vi "Write Report.vi"(8 "error in (no error)":errorcluster, 10 "Resource In":variant, 11 "Analyze Parameter Fluence in":refnum<class "Analyze Parameter Fluence.lvclass">) -> (0 "error out":errorcluster, 2 "Resource Out":variant, 3 "Analyze Parameter Fluence out":refnum<class "Analyze Parameter Fluence.lvclass">)   [LabVIEW 2014, in "Analyze Parameter Fluence.lvclass"]
uses:
  Analyze Parameter Fluence.lvclass
  Analyze Parameter Base/Analyze Parameter Base.lvclass
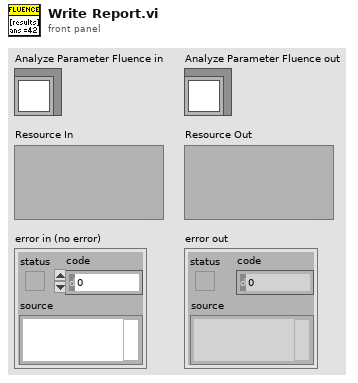
[diagram p1: front panel]
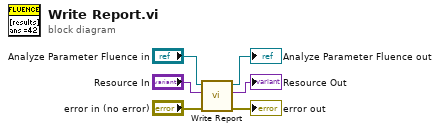
[diagram p0: block diagram]
diagram:
  n1 = call-parent "Write Report.vi"("error in (no error)"="error in (no error)", "Resource In"="Resource In", "Analyze Parameter Base in"="Analyze Parameter Fluence in") -> ("error out"=→"error out":errorcluster, "Resource Out"=→"Resource Out":variant, "Analyze Parameter Base out"=→"Analyze Parameter Fluence out":refnum<class "Analyze Parameter Fluence.lvclass">)  [unwired: 6 in]
